vi "fake resource short string.vi"(11 "input string":string) -> (3 "resulting string":string)   [LabVIEW 2025, in "MCP Server tests.lvlib"]
uses:
  MCP Server tests.lvlib
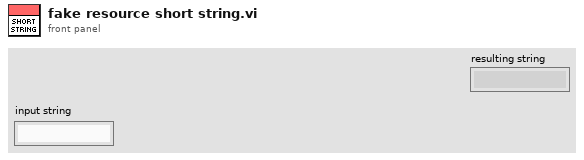
[diagram p1: front panel]
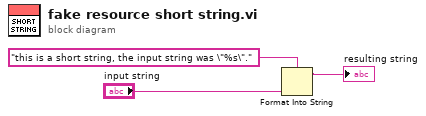
[diagram p0: block diagram]
diagram:
  n1 = Format Into String(format string="this is a short string, the input string was \"%s\".", "input string") -> (resulting string=→"resulting string":string)  [unwired: 2 in, 1 out]
